vi "Log_analyzer.vi"() -> ()   [LabVIEW 2023, in "Data Analysis.lvlib"]
uses:
  Data Analysis.lvlib
  HardwareAbstractionLayer_LVOOP/Database/SQL Public VI/Control/DB Options.ctl
  <vilib>/Utility/file.llb/Write Delimited Spreadsheet (string).vi
  HardwareAbstractionLayer_LVOOP/Database/Database.lvclass
panel:
  in  "Test Log":string(combo)
  in  "error in":errorcluster
  in  "Tab Control":T1(tab)=enum."Signal Analysis"
  in  "Test Info":i32(listbox)=-1 caption="Data"
  in  "Error Data":i32(listbox)=-1 caption="Data"
  in  "Error_Tree":string(tree) caption="Error Log"
  in  "Export Data( .csv)":bool
  in  "Reset Filters":bool
  in  "Filter Button Time":bool
  in  "Filter Button":bool
  in  "Test Mode":string(combo)
  in  "Stop Test Cycle":string(combo) caption="Test Cycle"
  in  "Start Test Cycle":string(combo) caption="Test Cycle"
  in  "Test Socket":string(combo)
  in  "Frame Type":string(combo)
  in  "Stop Time Stamp":timestamp format="%<%x %.3X>T"
  in  "Start Time Stamp":timestamp format="%<%x %.3X>T"
  in  "FE/FF Data":i32(listbox)=-1 caption="Data"
  out "XY Graph":cluster{dbl[], dbl[]}[](graph) caption="XY Graph - Dark"
  in  "Plot Signal":bool
  in  "Signal Name":string(combo)
  # "Data Filter"
  # "to"
  # "Time Based Filter"
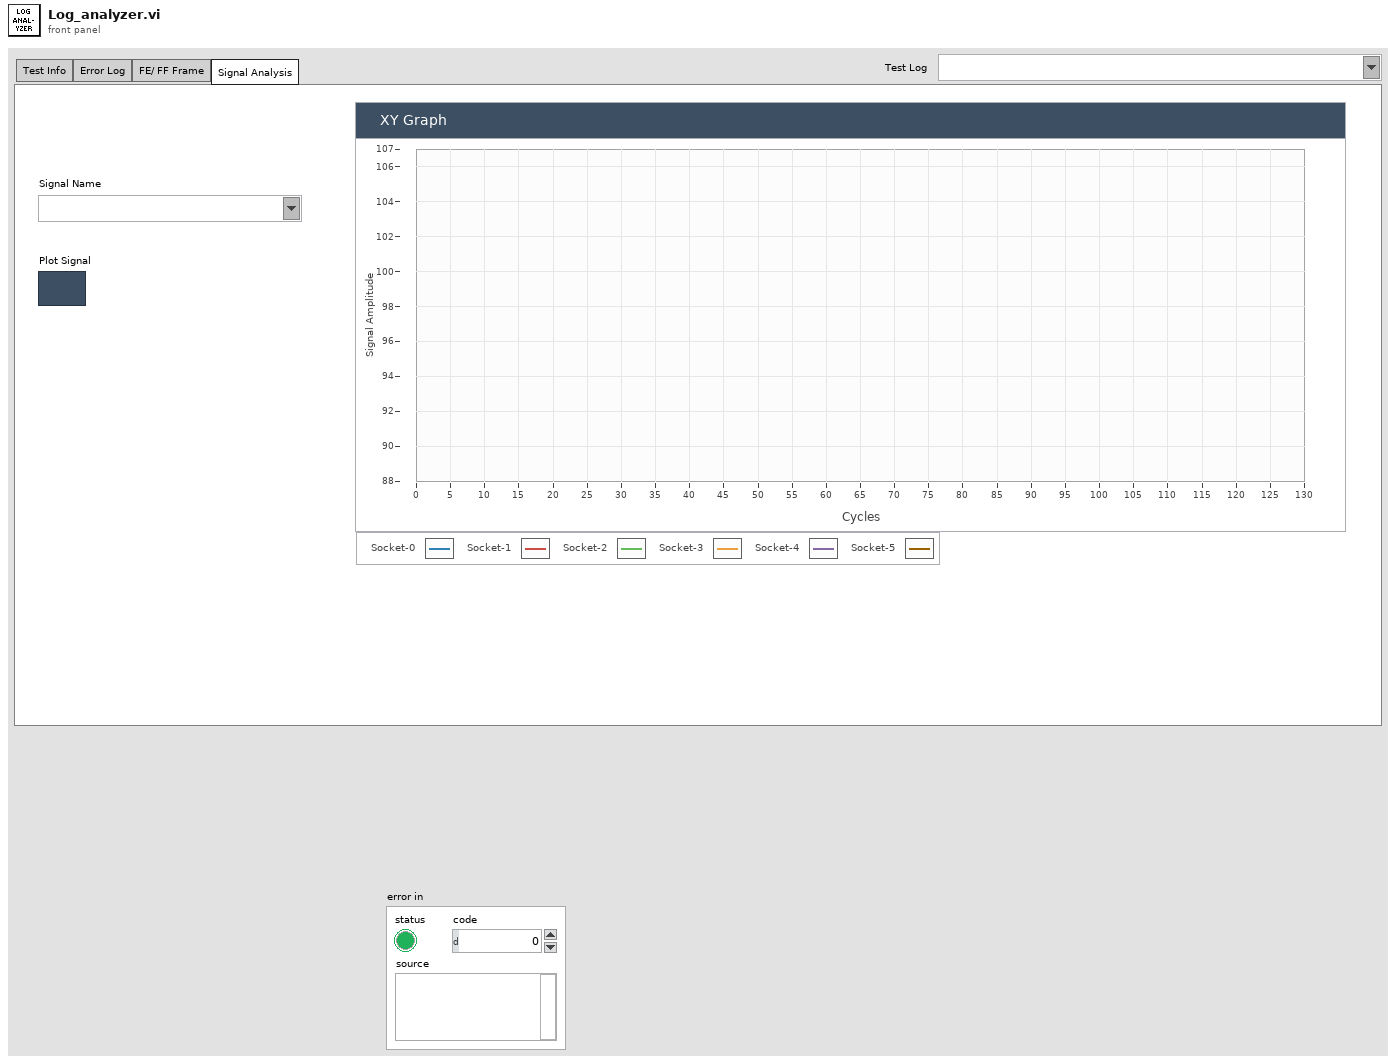
[diagram p1: front panel]
types:
  T1 = enum32{"Test Info", "Error Log", "FE/ FF Frame", "Signal Analysis"}
  T2 = typedef "HardwareAbstractionLayer_LVOOP.lvlib/Database.lvclass/DB Options.ctl" = enum16{"Init", "Select Data", "Insert Data", "Update Data", "Delete Data", "Execute Query", "Create Schema", "Create Table", "List Tables", "List Columns", "Close"}
  T3 = cluster{"table":string, "condition":string, "columns":string[]}
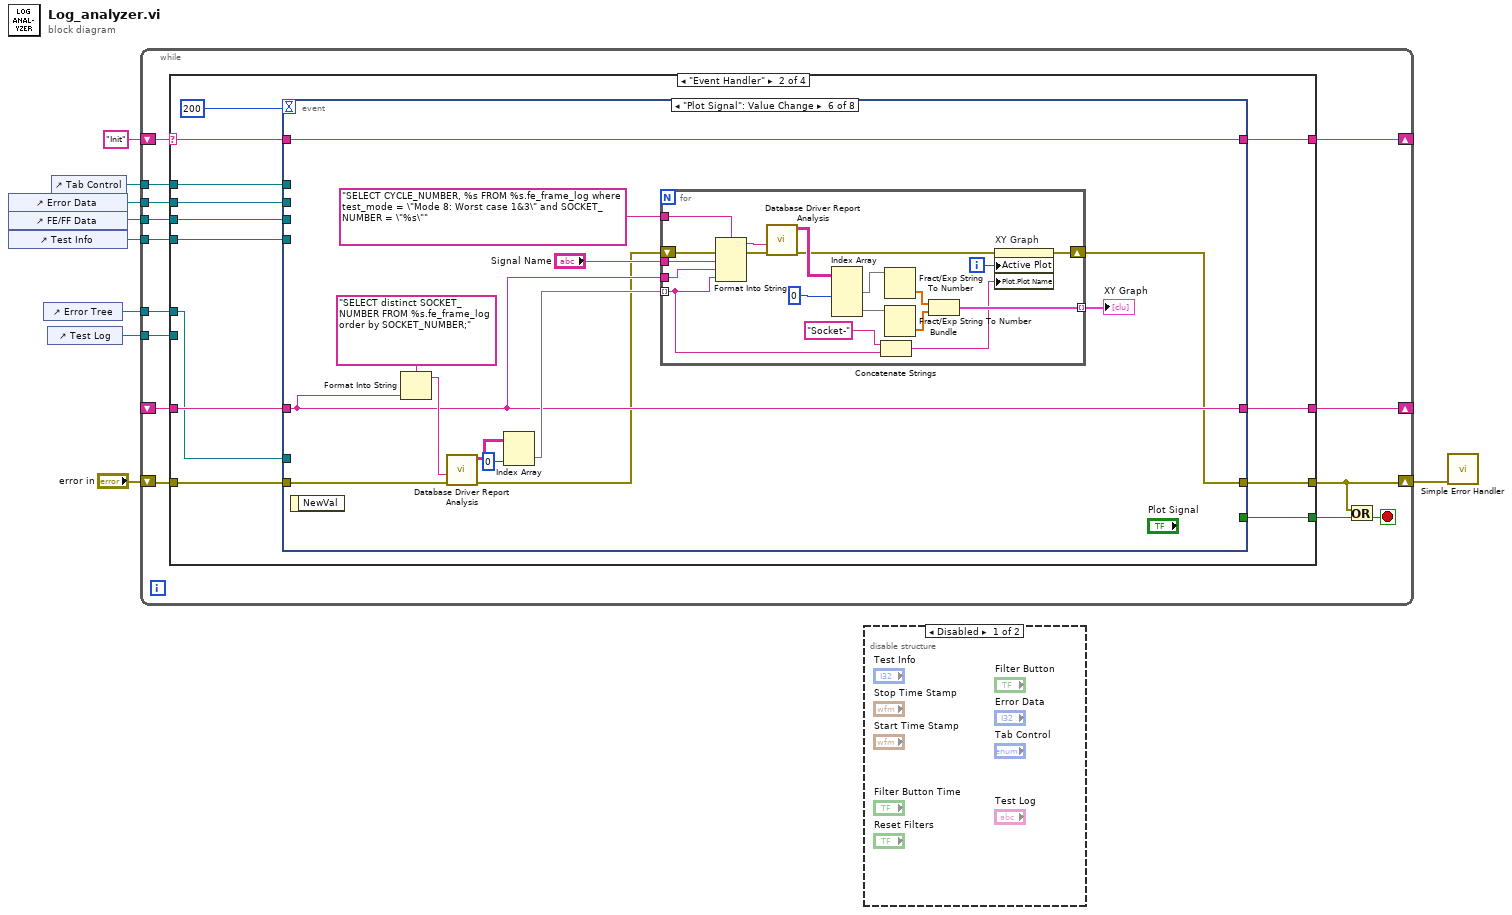
[diagram p0: block diagram]
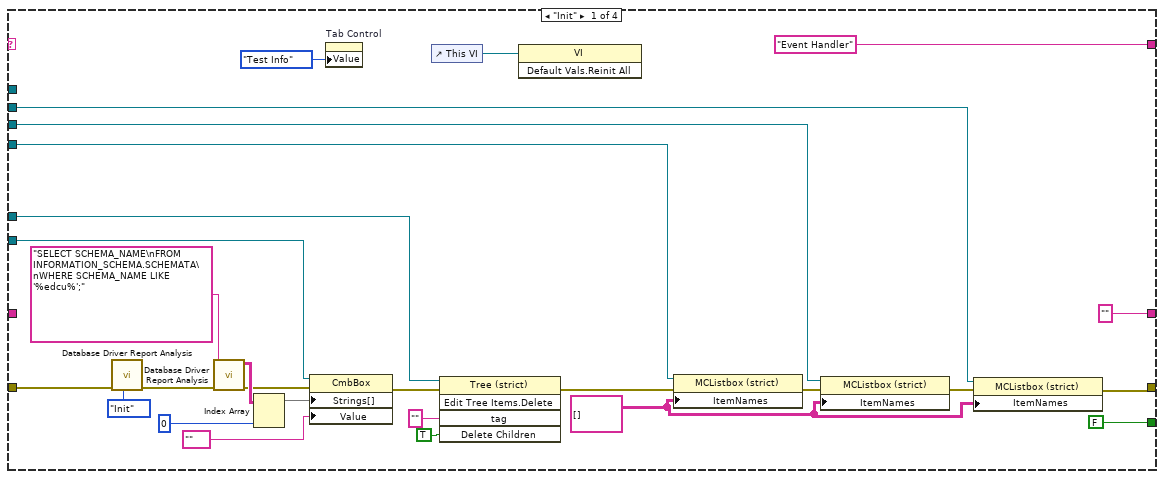
[diagram p2: hidden frame]
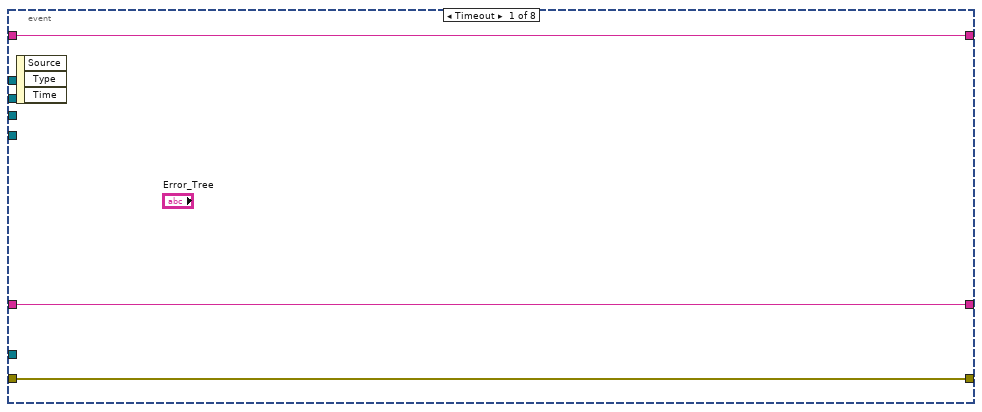
[diagram p3: hidden frame]
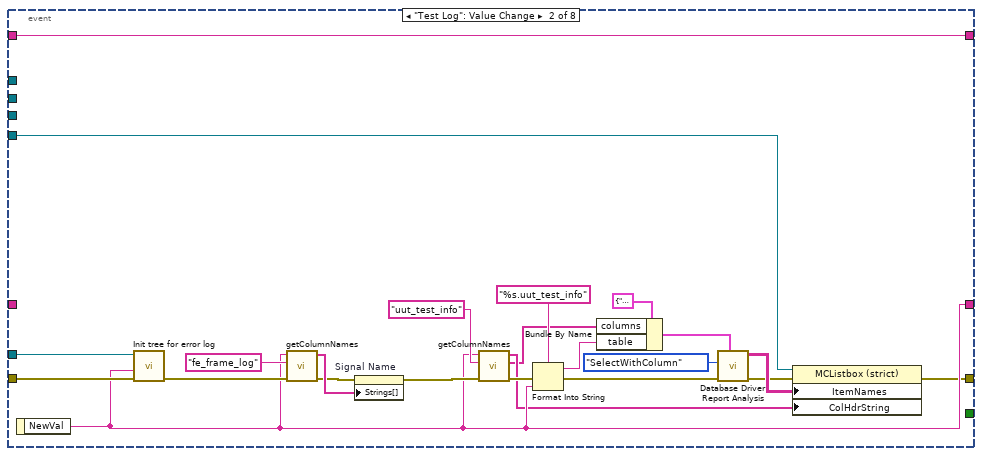
[diagram p4: hidden frame]
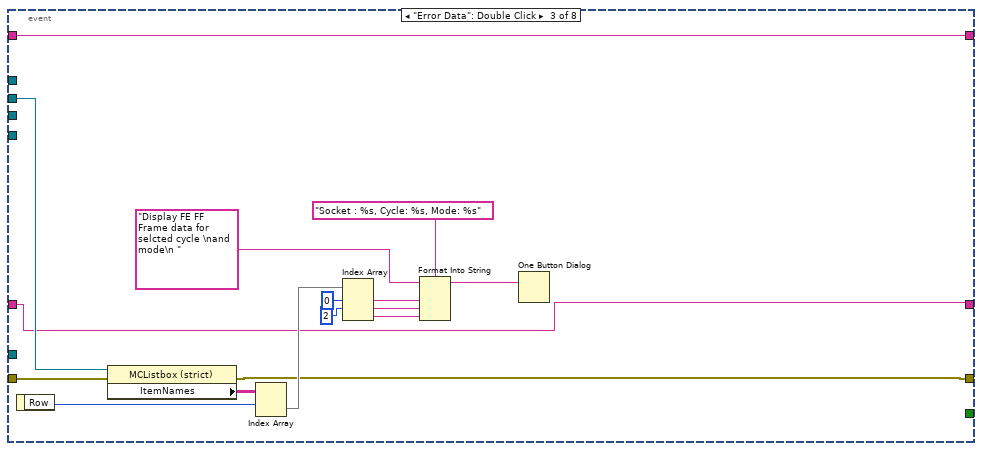
[diagram p5: hidden frame]
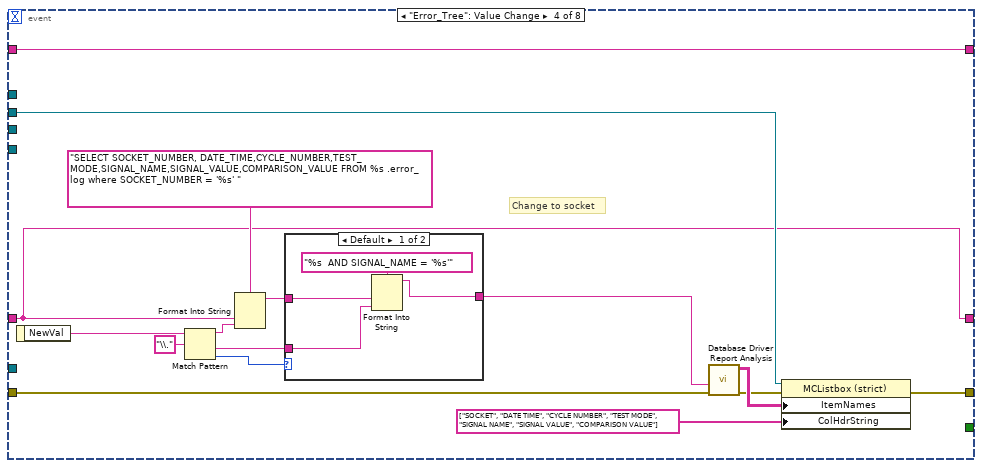
[diagram p6: hidden frame]
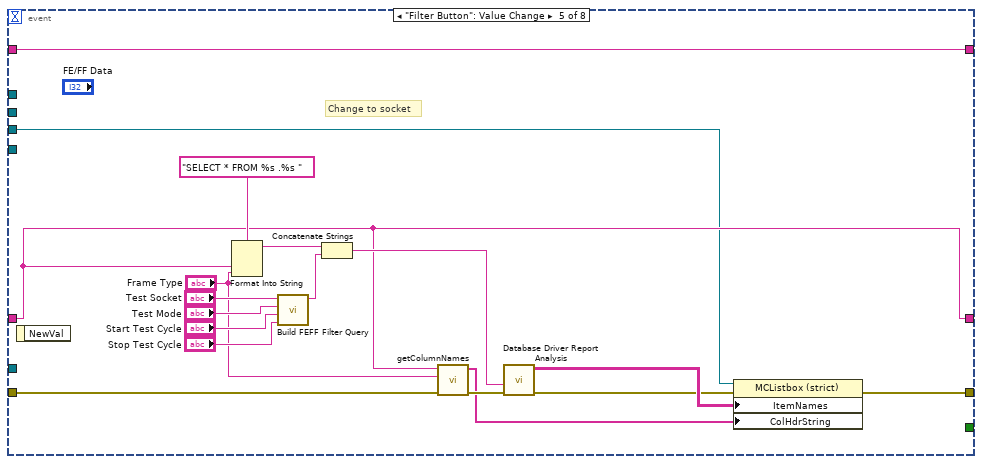
[diagram p8: hidden frame]
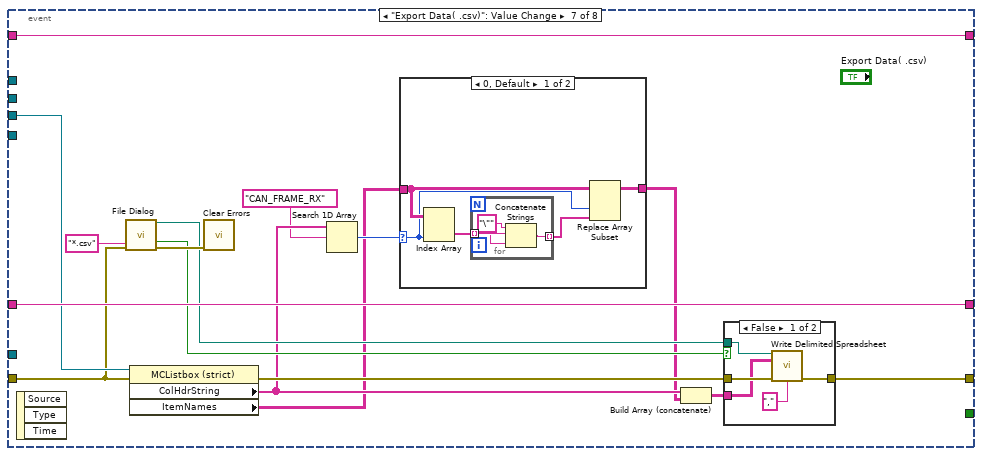
[diagram p9: hidden frame]
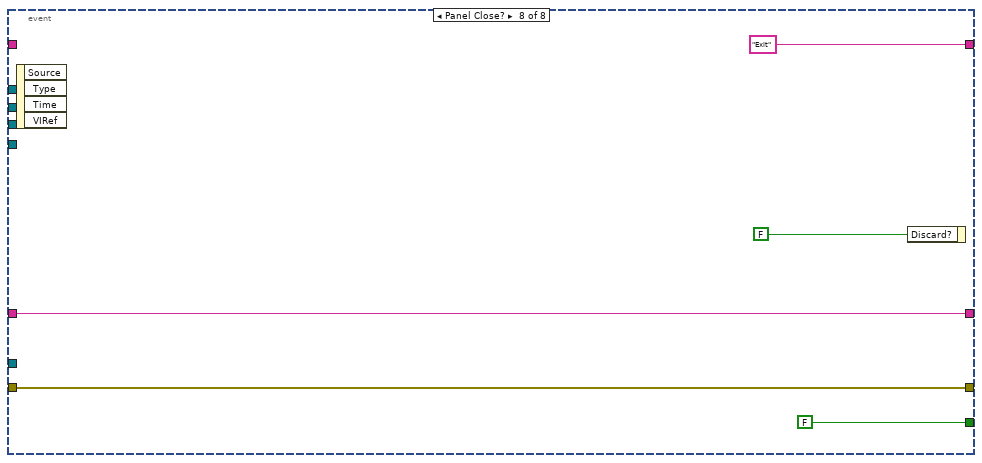
[diagram p12: hidden frame]
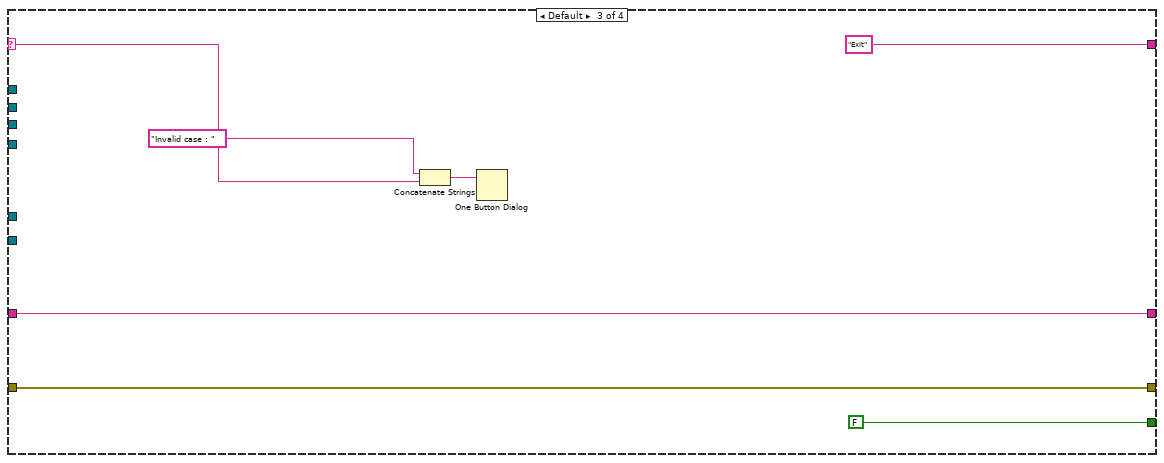
[diagram p13: hidden frame]
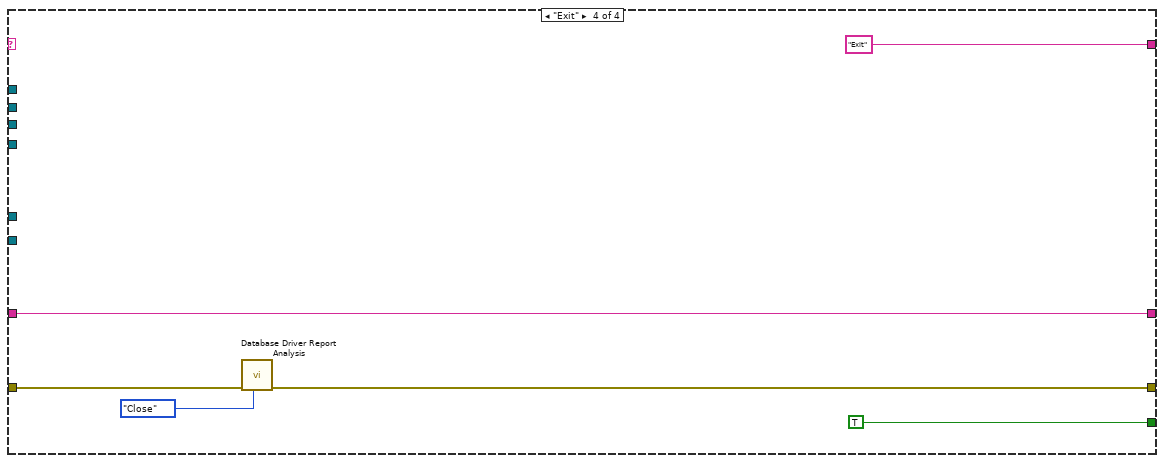
[diagram p14: hidden frame]
diagram:
  n1 = control-ref of="Error Data"() -> (w4:refnum<vi>)
  n2 = control-ref of="FE/FF Data"() -> (w2:refnum<vi>)
  n3 = control-ref of="Test Info"() -> (w1:refnum<vi>)
  n4 = control-ref of="Error Tree"() -> (w7:refnum<vi>)
  n5 = control-ref of="Test Log"() -> (w3:refnum<vi>)
  n6 = control-ref of="Tab Control"() -> (w6:refnum<vi>)
  n7 = while {
    shift-right: [w21] -> _
    shift-left: "Init" -> [w23]
    shift-right: [w12] -> w5
    shift-left: "error in" -> [w22]
    tunnel: w7 -> [w19]
    tunnel: w6 -> [w18]
    tunnel: w4 -> [w17]
    shift-right: [w15] -> _
    shift-left: _ -> [w16]
    tunnel: w3 -> [w14]
    tunnel: w2 -> [w11]
    tunnel: w1 -> [w10]
    stop <- w13 stop-if-true
    n8 = case shown="\"Event Handler\"" w23 {
      selector: w23 -> [_ w58 w216 _]
      tunnel: w22 -> [w49 w62 w219 w222]
      tunnel: [w29 w63 w219 w221] -> w12
      tunnel: ["Event Handler" w59 "Exit" "Exit"] -> w21
      tunnel: [FALSE w60 FALSE TRUE] -> w20
      tunnel: w19 -> [w39 w53 _ _]
      tunnel: w18 -> [_ w57 _ _]
      tunnel: w17 -> [w27 w56 _ _]
      tunnel: w16 -> [_ w55 w213 w220]
      tunnel: ["" ("NewVal") w54 w213 w220] -> w15
      tunnel: w14 -> [w35 _ _ _]
      tunnel: w11 -> [w26 w52 _ _]
      tunnel: w10 -> [w25 w51 _ _]
      frame "Init" {
        w28 = string[][] [] ("Item Names")
        n9 = call "Database Driver Report Analysis.vi"("Options"=DB_Options."Init", "error in"=w49) -> ("error out"=w46:errorcluster)  [unwired: 6 in, 3 out]
        n10 = call "Database Driver Report Analysis.vi"("error in"=w46, "SQL query"="SELECT SCHEMA_NAME\nFROM INFORMATION_SCHEMA.SCHEMATA\nWHERE SCHEMA_NAME LIKE '%edcu%';") -> ("error out"=w37:errorcluster, "data"=w44:string[][])  [unwired: 6 in, 2 out]
        n11 = Index Array(array=w44, index (col)=0 ("disabled index (col)")) -> (element=w34:string[])  [unwired: 1 in]
        n12 = property class="CmbBox"(reference=w35, error in=w37, "Strings[]"=w34, "Value"="" ("Test Log(Schema)")) -> (error out=w36:errorcluster)  [unwired: 1 out]
        n13 = property on="Tab Control" class="TabCtl (strict)"("Value"=T1."Test Info" ("Tab Control")) -> ()  [unwired: 2 in, 2 out]
        n14 = control-ref of="This VI"() -> (w32:refnum<vi>)
        n15 = invoke on="Invoke Node" class="Tree (strict)" method="Edit Tree Items.Delete"(reference=w39, error in=w36, "tag"="" ("Tag"), "Delete Children"=TRUE ("Delete Children?")) -> (error out=w38:errorcluster)  [unwired: 1 in, 4 out]
        n16 = invoke class="VI" method="Default Vals.Reinit All"(reference=w32) -> ()  [unwired: 2 in, 3 out]
        n17 = property class="MCListbox (strict)"(reference=w25, error in=w38, "ItemNames"=w28) -> (error out=w31:errorcluster)  [unwired: 1 out]
        n18 = property class="MCListbox (strict)"(reference=w26, error in=w31, "ItemNames"=w28) -> (error out=w30:errorcluster)  [unwired: 1 out]
        n19 = property class="MCListbox (strict)"(reference=w27, error in=w30, "ItemNames"=w28) -> (error out=w29:errorcluster)  [unwired: 1 out]
      }
      frame "Event Handler" {
        n20 = event shown="[5] \"Plot Signal\": Value Change" {
          selector: _ -> [_ _ _ _ _ _ _ _]
          dyn-events: _ -> [_ _ _ _ _ _ _ _]
          timeout: 200 -> [_ _ _ _ _ _ _ _]
          tunnel: [w66 w74 w91 w110 w139 w148 w188 w211] -> w63
          tunnel: w62 -> [w66 w88 w102 w108 w132 w156 w185 w211]
          tunnel: [_ _ _ _ _ _ _ FALSE] -> w60
          tunnel: [w65 w89 w105 w121 w144 w157 w192 "Exit"] -> w59
          tunnel: w58 -> [w65 w89 w105 w121 w144 w157 w192 _]
          tunnel: w55 -> [w64 _ w90 w107 w130 w149 w191 w208]
          tunnel: w57 -> [_ _ _ _ _ _ _ _]
          tunnel: w56 -> [_ _ w103 w113 _ _ _ _]
          tunnel: [w64 w78 w90 w107 w130 w149 w191 w208] -> w54
          tunnel: w53 -> [_ w87 _ _ _ _ _ _]
          tunnel: w52 -> [_ _ _ _ w127 _ w190 _]
          tunnel: w51 -> [_ w73 _ _ _ _ _ _]
          event Timeout {
            n21 = event-data() -> ()  [unwired: 1 in, 3 out]
          }
          event "Test Log": Value Change {
            n22 = event-data() -> ("NewVal"=w78:string)  [unwired: 1 in]
            n23 = call "Init tree for error log.vi"("error in (no error)"=w88, "Test Log(Schema)"=w78, "TreeControl in"=w87) -> ("error out"=w86:errorcluster)  [unwired: 8 in]
            n24 = call "getColumnNames.vi"("error in (no error)"=w86, "tableName"="fe_frame_log" ("schema"), "schema"=w78) -> ("error out"=w84:errorcluster, "columnNames"=w85:string[])  [unwired: 6 in, 1 out]
            n25 = property on="Signal Name" class="CmbBox"(error in=w84, "Strings[]"=w85) -> (error out=w81:errorcluster)  [unwired: 1 in, 1 out]
            n26 = call "getColumnNames.vi"("error in (no error)"=w81, "tableName"="uut_test_info" ("schema"), "schema"=w78) -> ("error out"=w80:errorcluster, "columnNamesForQuery"=w67:string[], "columnNames"=w68:string[])  [unwired: 6 in]
            n27 = Format Into String(format string="%s.uut_test_info" ("schema"), error in=w80, w78) -> (resulting string=w71:string, error out=w75:errorcluster)  [unwired: 1 in]
            n28 = Bundle By Name(cluster=T3 {"table"="", "condition"="", "columns"=[]} ("SQLTableData"), "columns"=w67, "table"=w71) -> (w70:T3)
            n29 = call "Database Driver Report Analysis.vi"("SQLTableData"=w70, "error in"=w75, "Select"=enum16{"SelectWithQuery", "SelectWithColumn"}."SelectWithColumn") -> ("error out"=w76:errorcluster, "data"=w77:string[][])  [unwired: 5 in, 2 out]
            n30 = property class="MCListbox (strict)"(reference=w73, error in=w76, "ItemNames"=w77, "ColHdrString"=w68) -> (error out=w74:errorcluster)  [unwired: 1 out]
          }
          event "Error Data": Double Click {
            n31 = event-data() -> ("Row"=w101:i32)  [unwired: 1 in]
            n32 = property class="MCListbox (strict)"(reference=w103, error in=w102) -> (error out=w91:errorcluster, "ItemNames"=w104:string[][])  [unwired: 1 out]
            n33 = Index Array(array=w104, index (row)=w101) -> (element=w100:string[])  [unwired: 1 in]
            n34 = Index Array(array=w100, index #1=0 ("index"), index #2=2 ("index")) -> (element #1=w96:string, element #2=w95:string, element #3=w94:string)  [unwired: 1 in]
            n35 = Format Into String(format string="Socket : %s, Cycle: %s, Mode: %s", initial string="Display FE FF Frame data for selcted cycle \nand mode\n " ("message"), w96, w95, w94) -> (resulting string=w92:string)  [unwired: 1 in, 1 out]
            n36 = One Button Dialog(message=w92) -> ()  [unwired: 1 in, 1 out]
          }
          event "Error_Tree": Value Change {
            # "Change to socket"
            n37 = event-data() -> ("NewVal"=w120:string)  [unwired: 1 in]
            n38 = Match Pattern(string=w120, regular expression="\\.") -> (before substring=w118:string, after substring=w109:string, offset past match=w115:i32)  [unwired: 1 in, 1 out]
            n39 = Format Into String(format string="SELECT SOCKET_NUMBER, DATE_TIME,CYCLE_NUMBER,TEST_MODE,SIGNAL_NAME,SIGNAL_VALUE,COMPARISON_VALUE FROM %s .error_log where SOCKET_NUMBER = '%s' " ("SQL query"), w107, w118) -> (resulting string=w117:string)  [unwired: 2 in, 1 out]
            n40 = case shown="Default" w115 {
              tunnel: w117 -> [w124 w126]
              tunnel: [w122 w126] -> w116
              tunnel: w109 -> [w123 _]
              frame Default {
                n41 = Format Into String(format string="%s  AND SIGNAL_NAME = '%s'" ("SQL query"), w124, w123) -> (resulting string=w122:string)  [unwired: 2 in, 1 out]
              }
              frame -1 {
              }
            }
            n42 = call "Database Driver Report Analysis.vi"("error in"=w108, "SQL query"=w116) -> ("error out"=w111:errorcluster, "data"=w112:string[][])  [unwired: 6 in, 2 out]
            n43 = property class="MCListbox (strict)"(reference=w113, error in=w111, "ItemNames"=w112, "ColHdrString"=string[] ["SOCKET", "DATE TIME", "CYCLE NUMBER", "TEST MODE", "SIGNAL NAME", "SIGNAL VALUE", "COMPARISON VALUE"] ("Column Header Strings[]")) -> (error out=w110:errorcluster)  [unwired: 1 out]
          }
          event "Filter Button": Value Change {
            # "Change to socket"
            n44 = event-data() -> ()  [unwired: 1 in, 1 out]
            n45 = Format Into String(format string="SELECT * FROM %s .%s " ("SQL query"), w130, "Frame Type") -> (resulting string=w143:string)  [unwired: 2 in, 1 out]
            n46 = call "Build FEFF Filter Query.vi"("Stop Test Cycle"="Stop Test Cycle", "Start Test Cycle"="Start Test Cycle", "Test Mode"="Test Mode", "Test Socket"="Test Socket") -> ("String"=w133:string)  [unwired: 7 in]
            n47 = Concatenate Strings(w143, w133) -> (w134:string)
            n48 = call "getColumnNames.vi"("error in (no error)"=w132, "tableName"="Frame Type", "schema"=w130) -> ("error out"=w131:errorcluster, "columnNames"=w128:string[])  [unwired: 6 in, 1 out]
            n49 = call "Database Driver Report Analysis.vi"("error in"=w131, "SQL query"=w134) -> ("error out"=w140:errorcluster, "data"=w141:string[][])  [unwired: 6 in, 2 out]
            n50 = property class="MCListbox (strict)"(reference=w127, error in=w140, "ItemNames"=w141, "ColHdrString"=w128) -> (error out=w139:errorcluster)  [unwired: 1 out]
          }
          event "Plot Signal": Value Change {
            n51 = event-data() -> ()  [unwired: 1 in, 1 out]
            n52 = Format Into String(format string="SELECT distinct SOCKET_NUMBER FROM %s.fe_frame_log order by SOCKET_NUMBER;", w149) -> (resulting string=w154:string)  [unwired: 2 in, 1 out]
            n53 = call "Database Driver Report Analysis.vi"("error in"=w156, "SQL query"=w154) -> ("error out"=w145:errorcluster, "data"=w153:string[][])  [unwired: 6 in, 2 out]
            n54 = Index Array(array=w153, index (col)=0 ("disabled index (col)")) -> (element=w152:string[])  [unwired: 1 in]
            n55 = for {
              tunnel: w152 -> [w159] mode=indexing
              tunnel: "SELECT CYCLE_NUMBER, %s FROM %s.fe_frame_log where test_mode = \"Mode 8: Worst case 1&3\" and SOCKET_NUMBER = \"%s\"" -> [w176]
              tunnel: "Signal Name" -> [w175]
              tunnel: w149 -> [w174]
              shift-right: [w163] -> w148
              shift-left: w145 -> [w171]
              tunnel: [w164] -> w147 mode=indexing
              i -> [w160]
              n56 = Format Into String(format string=w176, error in=w171, w175, w174, w159) -> (resulting string=w173:string, error out=w172:errorcluster)  [unwired: 1 in]
              n57 = call "Database Driver Report Analysis.vi"("error in"=w172, "SQL query"=w173) -> ("error out"=w162:errorcluster, "data"=w170:string[][])  [unwired: 6 in, 2 out]
              n58 = Index Array(array=w170, index (col) #1=0 ("disabled index (col)")) -> (element #1=w168:string[], element #2=w166:string[])  [unwired: 3 in]
              n59 = Concatenate Strings("Socket-" ("string"), w159) -> (w158:string)
              n60 = Fract/Exp String To Number(string=w168) -> (number=w167:dbl[])  [unwired: 3 in, 1 out]
              n61 = Fract/Exp String To Number(string=w166) -> (number=w165:dbl[])  [unwired: 3 in, 1 out]
              n62 = Bundle(w167, w165) -> (w164:cluster{dbl[], dbl[]})  [unwired: 1 in]
              n63 = property on="XY Graph" class="XYGraph (strict)"(error in=w162, "Active Plot"=w160, "Plot.Plot Name"=w158) -> (error out=w163:errorcluster)  [unwired: 1 in, 1 out]
            }
            "XY Graph" <- w147
          }
          event "Export Data( .csv)": Value Change {
            n64 = event-data() -> ()  [unwired: 1 in, 3 out]
            n65 = call "File Dialog"("error in"=w185, "pattern (all files)"="*.csv") -> ("selected path"=w182:path, "cancelled"=w184:bool, "error out"=w186:errorcluster)  [unwired: 10 in, 1 out]
            n66 = property class="MCListbox (strict)"(reference=w190, error in=w185) -> (error out=w189:errorcluster, "ColHdrString"=w181:string[], "ItemNames"=w178:string[][])  [unwired: 1 out]
            n67 = call <vilib>:"Clear Errors.vi"("error in (no error)"=w186) -> ()  [unwired: 5 in, 2 out]
            n68 = Search 1D Array(1D array=w181, element="CAN_FRAME_RX") -> (index of element=w179:i32)  [unwired: 1 in]
            n69 = case shown="0, Default" w179 {
              selector: w179 -> [w194 _]
              tunnel: w178 -> [w196 w201]
              tunnel: [w195 w201] -> w177
              frame 0, Default {
                n70 = Index Array(array=w196, index (col)=w194) -> (element=w197:string[])  [unwired: 1 in]
                n71 = for {
                  tunnel: w197 -> [w200] mode=indexing
                  tunnel: [w198] -> w193 mode=indexing
                  w199 = "\""
                  n72 = Concatenate Strings(w199, w200, w199) -> (w198:string)
                }
                n73 = Replace Array Subset(array=w196, new element=w193, index (col)=w194) -> (w195:string[][])  [unwired: 1 in]
              }
              frame -1 {
              }
            }
            n74 = Build Array (concatenate)(w181, w177) -> (w183:string[][])
            n75 = case shown="False" w184 {
              tunnel: w189 -> [w206 w207]
              tunnel: [w205 w207] -> w188
              tunnel: w183 -> [w204 _]
              tunnel: w182 -> [w203 _]
              frame False {
                n76 = call-poly <vilib>:"Write Delimited Spreadsheet.vi"("file path (dialog if empty)"=w203, "2D data"=w204, "error in (no error)"=w206, "delimiter (\\t)"="," ("delimiter (\\t)")) -> ("error out"=w205:errorcluster)  [unwired: 10 in, 1 out]
              }
              frame True {
              }
            }
          }
          event Panel Close? {
            n77 = event-data() -> ()  [unwired: 1 in, 4 out]
            n78 = event-data("Discard?"=FALSE) -> ()  [unwired: 1 in, 1 out]
          }
        }
      }
      frame Default {
        n79 = Concatenate Strings("Invalid case : " ("string"), w216) -> (w214:string)
        n80 = One Button Dialog(message=w214) -> ()  [unwired: 1 in, 1 out]
      }
      frame "Exit" {
        n81 = call "Database Driver Report Analysis.vi"("Options"=DB_Options."Close", "error in"=w222) -> ("error out"=w221:errorcluster)  [unwired: 6 in, 3 out]
      }
    }
    n82 = Or(x=w12, y=w20) -> (x .or. y?=w13:bool)
  }
  n83 = disable-structure shown="Disabled" {
    frame Disabled {
    }
    frame Enabled {
    }
  }
  n84 = call <vilib>:"Simple Error Handler.vi"("error in (no error)"=w5) -> ()  [unwired: 4 in, 5 out]
